vi "Punkt koncowy widocznosci.vi"(7 "Kierunek":i16, 8 "error in (no error)":errorcluster, 10 "Start Pos":T1, 11 "Percepcja":cluster{"Zakres":i16, "Kat":i16}={"Zakres"=30, "Kat"=120}) -> (0 "error out":errorcluster, 2 "Final Pos":T1)   [LabVIEW 2014, in "Swiat.lvclass"]
uses:
  Swiat.lvclass
  Typedefs/Position.ctl
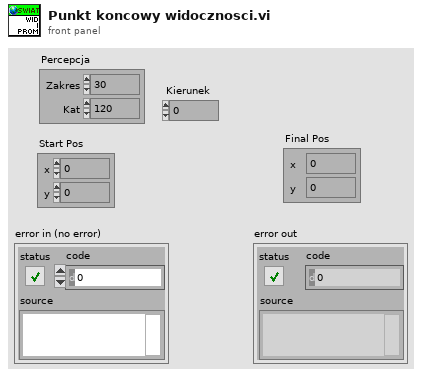
[diagram p1: front panel]
types:
  T1 = typedef "Position.ctl" = cluster{"x":i16, "y":i16}
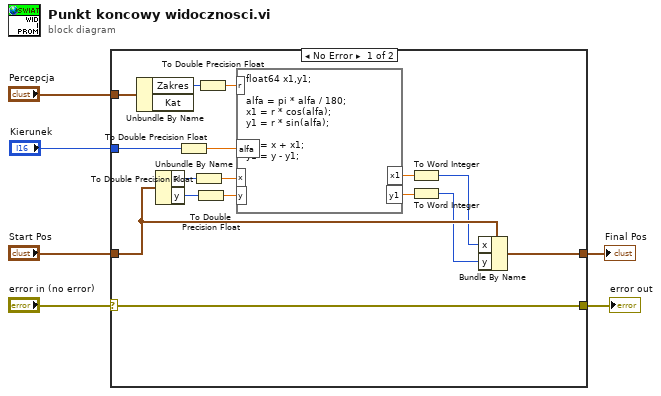
[diagram p0: block diagram]
diagram:
  n1 = case shown="No Error" "error in (no error)" {
    selector: "error in (no error)" -> [w22 w24]
    tunnel: [w22 w24] -> w5
    tunnel: [w19 w23] -> w4
    tunnel: "Start Pos" -> [w18 w23]
    tunnel: "Percepcja" -> [w21 _]
    tunnel: "Kierunek" -> [w17 _]
    frame No Error {
      n2 = Unbundle By Name(w21) -> ("Zakres"=w20:i16)  [unwired: 1 out]
      n3 = Unbundle By Name(w18) -> ("x"=w14:i16, "y"=w13:i16)
      n4 = To Double Precision Float(number=w17) -> (double precision float=w15:dbl)
      n5 = To Double Precision Float(number=w14) -> (double precision float=w12:dbl)
      n6 = To Double Precision Float(number=w13) -> (double precision float=w11:dbl)
      n7 = To Double Precision Float(number=w20) -> (double precision float=w16:dbl)
      n8 = formula code="float64 x1,y1;\n\nalfa = pi * alfa / 180;\nx1 = r * cos(alfa);\ny1 = r * sin(alfa);\n\nx1 = x + x1;\ny1 = y - y1;"("r"=w16, "alfa"=w15, "x"=w12, "y"=w11) -> ("x1"=w10:dbl, "y1"=w9:dbl)
      n9 = To Word Integer(number=w10) -> (16bit integer=w7:i16)
      n10 = To Word Integer(number=w9) -> (16bit integer=w8:i16)
      n11 = Bundle By Name(cluster=w18, "x"=w7, "y"=w8) -> (w19:T1)
    }
    frame Error {
    }
  }
  "Final Pos" <- w4
  "error out" <- w5
